vi "Default Instrument Setup.vi"(8 "error in (no error)":errorcluster, 11 "VISA resource name":refnum<visa-resource-name>) -> (0 "error out":errorcluster, 3 "VISA resource name out":refnum<visa-resource-name>)   [LabVIEW 2019, in "Keithley 2600 Series.lvlib"]
doc: "Sends a default command string to the instrument whenever a new VISA session is opened, or the instrument is reset. Use this VI as a subVI for the <b>Initialize</b> and <b>Reset</b> VIs. Altering this VI could cause these two VIs to operate incorrectly."
uses:
  Keithley 2600 Series.lvlib
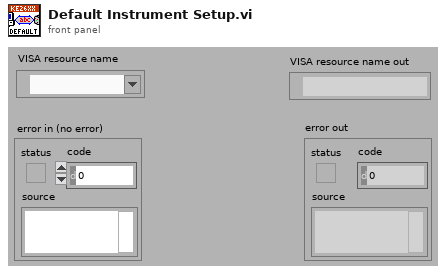
[diagram p1: front panel]
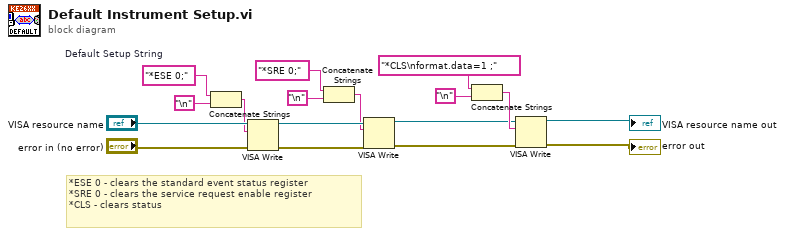
[diagram p0: block diagram]
diagram:
  w14 = "*ESE 0;"  # Default Setup String
  # "*ESE 0 - clears the standard event status register\n*SRE 0 - clears the service request enable register\n*CLS - clears status"
  n1 = Concatenate Strings(w14, "\n") -> (w9:string)
  n2 = VISA Write(VISA resource name="VISA resource name", write buffer=w9, error in (no error)="error in (no error)") -> (VISA resource name out=w7:refnum<visa-resource-name>, error out=w4:errorcluster)  [unwired: 1 out]
  n3 = Concatenate Strings("*SRE 0;", "\n") -> (w1:string)
  n4 = VISA Write(VISA resource name=w7, write buffer=w1, error in (no error)=w4) -> (VISA resource name out=w6:refnum<visa-resource-name>, error out=w2:errorcluster)  [unwired: 1 out]
  n5 = Concatenate Strings("*CLS\nformat.data=1 ;", "\n") -> (w8:string)
  n6 = VISA Write(VISA resource name=w6, write buffer=w8, error in (no error)=w2) -> (VISA resource name out=→"VISA resource name out":refnum<visa-resource-name>, error out=→"error out":errorcluster)  [unwired: 1 out]
